vi "ConvertXY.vi"(10 "흥분도(Y)":dbl, 11 "행복도(X)":dbl) -> (3 "Color":u32[](array[colorbox]))   [LabVIEW 2020]
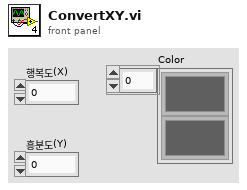
[diagram p1: front panel]
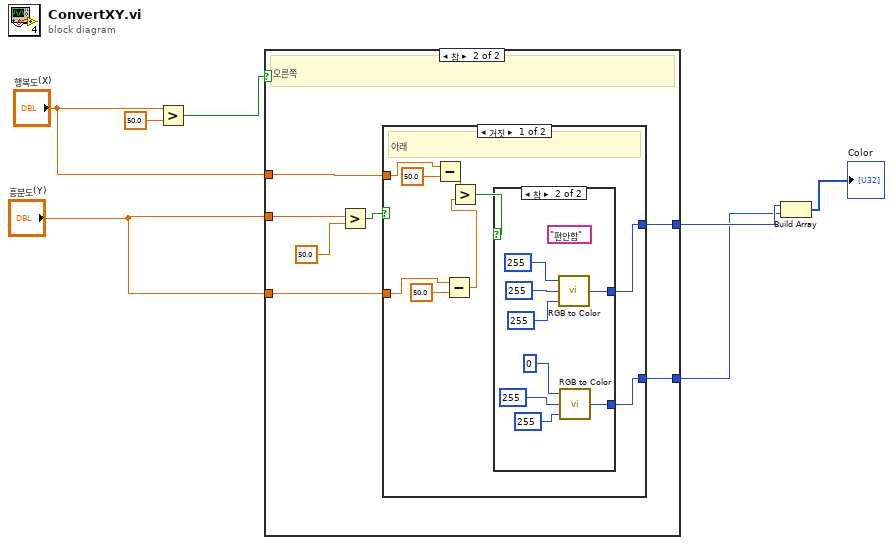
[diagram p0: block diagram]
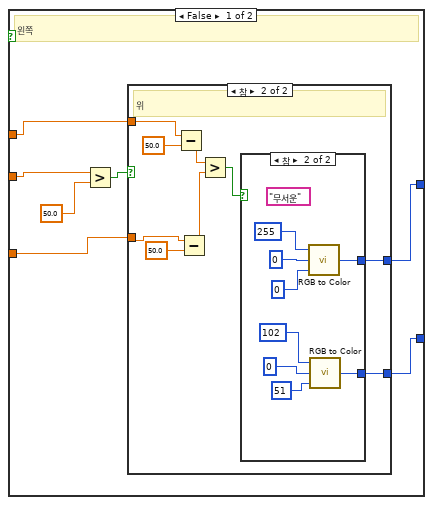
[diagram p2: hidden frame]
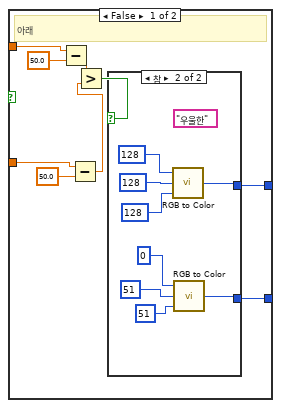
[diagram p3: hidden frame]
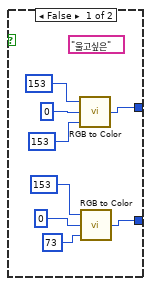
[diagram p4: hidden frame]
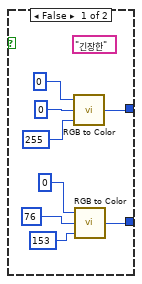
[diagram p5: hidden frame]
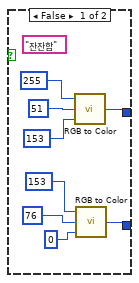
[diagram p6: hidden frame]
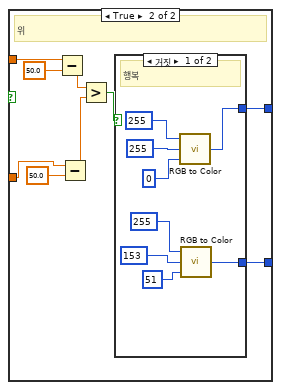
[diagram p7: hidden frame]
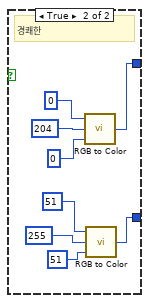
[diagram p8: hidden frame]
diagram:
  n1 = Greater?(x="행복도(X)", y=50.0) -> (0:w6:bool)
  n2 = case shown="참" w6 {
    tunnel: "흥분도(Y)" -> [w11 w70]
    tunnel: "행복도(X)" -> [w12 w68]
    tunnel: "흥분도(Y)" -> [w10 w67]
    tunnel: [w9 w66] -> w3
    tunnel: [w8 w65] -> w2
    frame False {
      # "왼쪽"
      n3 = Greater?(x=w11, y=50.0) -> (0:w13:bool)
      n4 = case shown="참" w13 {
        tunnel: w12 -> [w18 w43]
        tunnel: w10 -> [w17 w42]
        tunnel: [w16 w41] -> w9
        tunnel: [w15 w40] -> w8
        frame False {
          # "아래"
          n5 = Subtract(x=w18, y=50.0) -> (x-y=w21:dbl)
          n6 = Subtract(x=w17, y=50.0) -> (x-y=w19:dbl)
          n7 = Greater?(x=w21, y=w19) -> (0:w23:bool)
          n8 = case shown="참" w23 {
            tunnel: [w25 w33] -> w16
            tunnel: [w24 w32] -> w15
            frame False {
              (unwired) "울고싶은"
              n9 = call <vilib>:"RGB to Color.vi"("B"=u8 153, "G"=u8 0, "R"=u8 153) -> ("Color"=w25:u32)
              n10 = call <vilib>:"RGB to Color.vi"("B"=u8 73, "G"=u8 0, "R"=u8 153) -> ("Color"=w24:u32)
            }
            frame True {
              (unwired) "우울한"
              n11 = call <vilib>:"RGB to Color.vi"("B"=u8 128, "G"=u8 128, "R"=u8 128) -> ("Color"=w33:u32)
              n12 = call <vilib>:"RGB to Color.vi"("B"=u8 51, "G"=u8 51, "R"=u8 0) -> ("Color"=w32:u32)
            }
          }
        }
        frame True {
          # "위"
          n13 = Subtract(x=w43, y=50.0) -> (x-y=w47:dbl)
          n14 = Subtract(x=w42, y=50.0) -> (x-y=w44:dbl)
          n15 = Greater?(x=w47, y=w44) -> (0:w48:bool)
          n16 = case shown="참" w48 {
            tunnel: [w50 w58] -> w41
            tunnel: [w49 w57] -> w40
            frame False {
              (unwired) "긴장한"
              n17 = call <vilib>:"RGB to Color.vi"("B"=u8 255, "G"=u8 0, "R"=u8 0) -> ("Color"=w50:u32)
              n18 = call <vilib>:"RGB to Color.vi"("B"=u8 153, "G"=u8 76, "R"=u8 0) -> ("Color"=w49:u32)
            }
            frame True {
              (unwired) "무서운"
              n19 = call <vilib>:"RGB to Color.vi"("B"=u8 0, "G"=u8 0, "R"=u8 255) -> ("Color"=w58:u32)
              n20 = call <vilib>:"RGB to Color.vi"("B"=u8 51, "G"=u8 0, "R"=u8 102) -> ("Color"=w57:u32)
            }
          }
        }
      }
    }
    frame True {
      # "오른쪽"
      n21 = Greater?(x=w70, y=50.0) -> (0:w69:bool)
      n22 = case shown="거짓" w69 {
        tunnel: w68 -> [w79 w103]
        tunnel: w67 -> [w76 w101]
        tunnel: [w73 w98] -> w66
        tunnel: [w72 w97] -> w65
        frame False {
          # "아래"
          n23 = Subtract(x=w79, y=50.0) -> (x-y=w77:dbl)
          n24 = Subtract(x=w76, y=50.0) -> (x-y=w74:dbl)
          n25 = Greater?(x=w77, y=w74) -> (0:w80:bool)
          n26 = case shown="참" w80 {
            tunnel: [w82 w90] -> w73
            tunnel: [w81 w89] -> w72
            frame False {
              (unwired) "잔잔함"
              n27 = call <vilib>:"RGB to Color.vi"("B"=u8 153, "G"=u8 51, "R"=u8 255) -> ("Color"=w82:u32)
              n28 = call <vilib>:"RGB to Color.vi"("B"=u8 0, "G"=u8 76, "R"=u8 153) -> ("Color"=w81:u32)
            }
            frame True {
              (unwired) "편안함"
              n29 = call <vilib>:"RGB to Color.vi"("B"=u8 255, "G"=u8 255, "R"=u8 255) -> ("Color"=w90:u32)
              n30 = call <vilib>:"RGB to Color.vi"("B"=u8 255, "G"=u8 255, "R"=u8 0) -> ("Color"=w89:u32)
            }
          }
        }
        frame True {
          # "위"
          n31 = Subtract(x=w103, y=50.0) -> (x-y=w104:dbl)
          n32 = Subtract(x=w101, y=50.0) -> (x-y=w99:dbl)
          n33 = Greater?(x=w104, y=w99) -> (0:w105:bool)
          n34 = case shown="거짓" w105 {
            tunnel: [w107 w115] -> w98
            tunnel: [w106 w114] -> w97
            frame False {
              # "행복"
              n35 = call <vilib>:"RGB to Color.vi"("B"=u8 0, "G"=u8 255, "R"=u8 255) -> ("Color"=w107:u32)
              n36 = call <vilib>:"RGB to Color.vi"("B"=u8 51, "G"=u8 153, "R"=u8 255) -> ("Color"=w106:u32)
            }
            frame True {
              # "경쾌한"
              n37 = call <vilib>:"RGB to Color.vi"("B"=u8 0, "G"=u8 204, "R"=u8 0) -> ("Color"=w115:u32)
              n38 = call <vilib>:"RGB to Color.vi"("B"=u8 51, "G"=u8 255, "R"=u8 51) -> ("Color"=w114:u32)
            }
          }
        }
      }
    }
  }
  n39 = Build Array(w3, w2) -> (→"Color":u32[])
